vi "getsn_web.vi"(3 "strDate":string, 4 "sSN":string, 5 "strPartNo":string) -> (0 "error out":errorcluster caption="错误输出", 1 "strErrMsg":string, 2 "getCode":string[](array[string]))   [LabVIEW 2011]
uses:
  <vilib>/Utility/xml.llb/Write to XML File(string).vi
  <vilib>/Utility/xml.llb/Read From XML File(string).vi
panel:
  in  ".NET:EEPromCodeService.ParaClass":T1
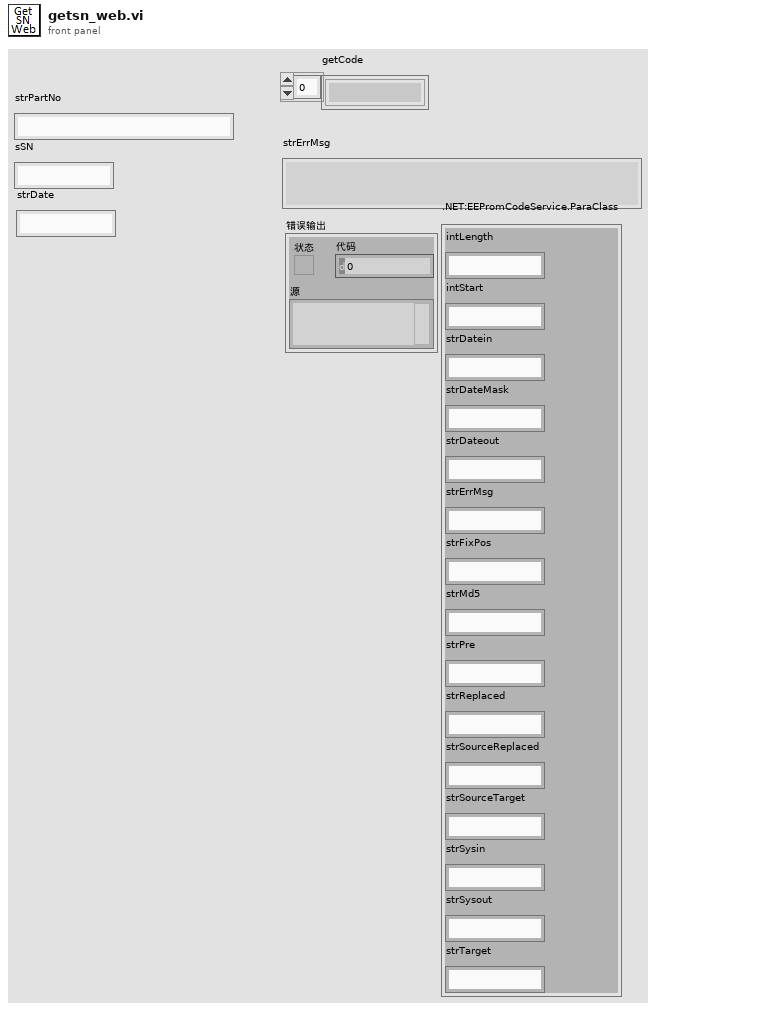
[diagram p1: front panel]
types:
  T1 = cluster{"intLength":string, "intStart":string, "strDatein":string, "strDateMask":string, "strDateout":string, "strErrMsg":string, "strFixPos":string, "strMd5":string, "strPre":string, "strReplaced":string, "strSourceReplaced":string, "strSourceTarget":string, "strSysin":string, "strSysout":string, "strTarget":string}
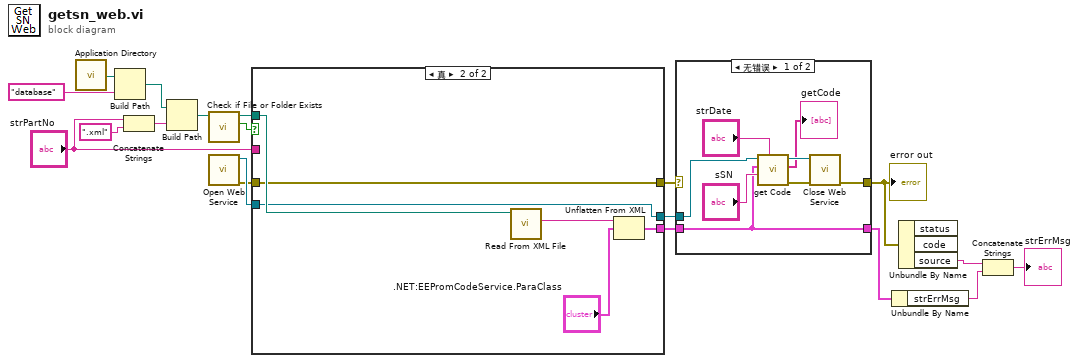
[diagram p0: block diagram]
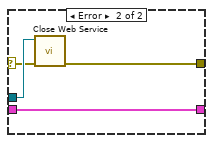
[diagram p2: hidden frame]
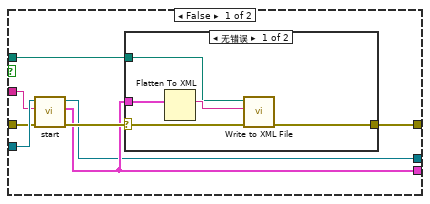
[diagram p3: hidden frame]
diagram:
  n1 = call <vilib>:"Application Directory.vi"() -> ("Application Directory"=w19:path)
  n2 = Build Path(base path=w19, name or relative path="database" ("名称或相对路径")) -> (appended path=w17:path)
  n3 = Concatenate Strings("strPartNo", ".xml" ("字符串")) -> (w15:string)
  n4 = Build Path(base path=w17, name or relative path=w15) -> (appended path=w14:path)
  n5 = call <vilib>:"Check if File or Folder Exists.vi"("path"=w14) -> ("file or folder exists?"=w13:bool, "dup path"=w12:path)  [unwired: 8 in, 1 out]
  n6 = call "Open Web Service.vi"() -> ("error out"=w10:errorcluster, "EEPromCodeService 引用句柄"=w11:refnum<k24>)  [unwired: 10 in]
  n7 = case shown="真" w13 {
    tunnel: w12 -> [w21 w39]
    tunnel: w11 -> [w27 w35]
    tunnel: w10 -> [w25 w34]
    tunnel: "strPartNo" -> [w26 _]
    tunnel: [w23 w36] -> w8
    tunnel: [w22 w35] -> w7
    tunnel: [w20 w34] -> w6
    frame False {
      n8 = call "start.vi"("error in (no error)"=w25, "strPartNo"=w26, "EEPromCodeService 引用句柄"=w27) -> ("error out"=w24:errorcluster, ".NET:EEPromCodeService.ParaClass"=w23:T1, "EEPromCodeService 引用句柄输出"=w22:refnum<k24>)  [unwired: 6 in]
      n9 = case shown="无错误" w24 {
        selector: w24 -> [w29 w33]
        tunnel: w23 -> [w31 _]
        tunnel: w21 -> [w30 _]
        tunnel: [w28 w33] -> w20
        frame No Error {
          n10 = Flatten To XML(anything=w31) -> (xml string=w32:string)
          n11 = call-poly <vilib>:"Write to XML File.vi"("error in (no error)"=w29, "XML Input"=w32, "XML File Path"=w30) -> ("error out"=w28:errorcluster)  [unwired: 6 in, 2 out]
        }
        frame Error {
        }
      }
    }
    frame True {
      n12 = call-poly <vilib>:"Read From XML File.vi"("XML File Path"=w39) -> ("XML Elements"=w38:string)  [unwired: 8 in, 2 out]
      n13 = Unflatten From XML(xml string=w38, type=".NET:EEPromCodeService.ParaClass") -> (value=w36:T1)  [unwired: 1 in, 1 out]
    }
  }
  n14 = case shown="无错误" w6 {
    selector: w6 -> [_ w50]
    tunnel: w8 -> [w40 w48]
    tunnel: w7 -> [w42 w51]
    tunnel: [w41 w49] -> w1
    tunnel: [w40 w48] -> w2
    frame No Error {
      n15 = call "get Code.vi"("strDate"="strDate", "sSN"="sSN", ".NET:EEPromCodeService.ParaClass"=w40, "EEPromCodeService 引用句柄"=w42) -> ("error out"=w43:errorcluster, "getCode"=→"getCode":string[], "EEPromCodeService 引用句柄输出"=w45:refnum<k24>)  [unwired: 5 in]
      n16 = call "Close Web Service.vi"("error in (no error)"=w43, "EEPromCodeService 引用句柄"=w45) -> ("error out"=w41:errorcluster)  [unwired: 9 in]
    }
    frame Error {
      n17 = call "Close Web Service.vi"("error in (no error)"=w50, "EEPromCodeService 引用句柄"=w51) -> ("error out"=w49:errorcluster)  [unwired: 9 in]
    }
  }
  "error out" <- w1
  n18 = Unbundle By Name(w2) -> ("strErrMsg"=w4:string)
  n19 = Unbundle By Name(w1) -> ("source"=w3:string)  [unwired: 2 out]
  n20 = Concatenate Strings(w3, w4) -> (→"strErrMsg":string)
